vi "Actor Core.vi"(8 "error in":errorcluster, 11 "Nested in":refnum<class "UI Actor.lvclass">) -> (0 "error out":errorcluster, 3 "Actor out":refnum<class "Actor.lvclass">)   [LabVIEW 2020, in "UI Actor.lvlib" / "UI Actor.lvclass"]
doc: "(<B>Filename</B>: Actor Framework.lvlib:Actor.lvclass:Actor Core.vi)\n\nReceives messages to the actor, reacts to them, and initiates any error handling that may shut the actor down.\n\nDescendant classes may override this VI to append parallel tasks for the actor to complete while it handles messages. Overrides use the Call Parent Method node."
uses:
  UI Actor.lvclass
  <vilib>/ActorFramework/Actor/Actor.lvclass
  <vilib>/ActorFramework/Stop Msg/Stop Msg.lvclass
  Sub Panel Actor.lvclass
  C:/Program Files (x86)/National Instruments/LabVIEW 2020/vi.lib/ActorFramework/Actor/Actor.lvclass
  C:/Users/eddiews/Documents/Git Hub Repositorios/VendingMachine_ActorFramework/UI Actor.lvclass
  C:/Users/eddiews/Documents/Git Hub Repositorios/VendingMachine_ActorFramework/Sub Panel Actor.lvclass
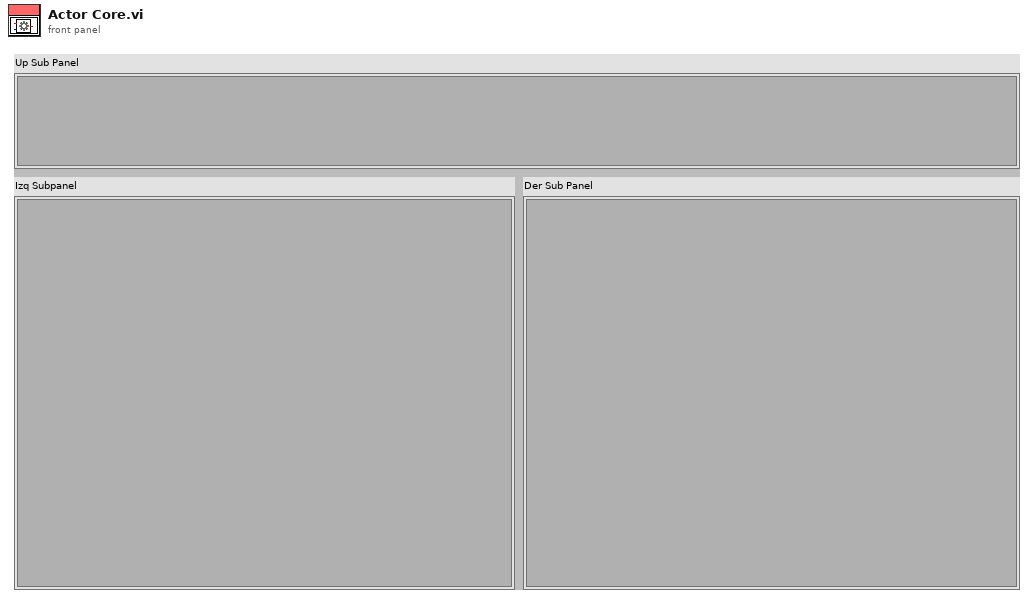
[diagram p1: front panel]
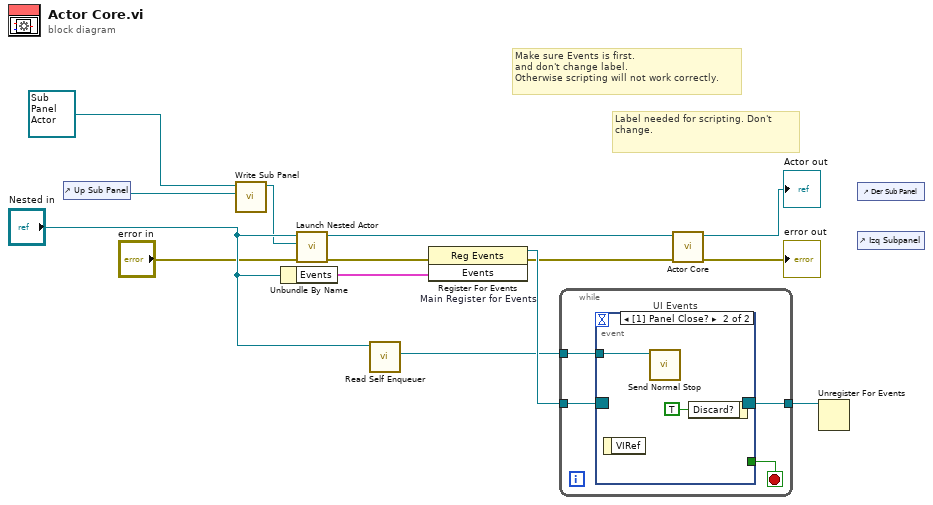
[diagram p0: block diagram]
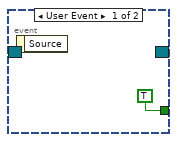
[diagram p2: hidden frame]
diagram:
  # "Label needed for scripting. Don't change."
  # "Make sure Events is first.\nand don't change label.\nOtherwise scripting will not work correctly."
  n1 = control-ref of="Up Sub Panel"() -> (w1:refnum<vi>)
  n2 = call "Write Sub Panel.vi"("Sub Panel"=w1, "Sub Panel Actor in"=refnum<class "Sub Panel Actor.lvclass"> refnum ("Sub Panel Actor.lvlib:Sub Panel Actor.lvclass")) -> ("Sub Panel Actor out"=w4:refnum<class "Sub Panel Actor.lvclass">)  [unwired: 8 in, 1 out]
  n3 = Unbundle By Name("Nested in") -> ("Events"=w11:cluster{"Stop":refnum<user-event>})
  n4 = call <vilib>:"Launch Nested Actor.vi"("error in (no error)"="error in", "Nested Actor"=w4, "Caller Actor in"="Nested in") -> ("error out"=w3:errorcluster, "Caller Actor out"=w6:refnum<class "UI Actor.lvclass">)  [unwired: 6 in, 1 out]
  n5 = call <vilib>:"Read Self Enqueuer.vi"("Actor"="Nested in") -> ("Self Enqueuer"=w9:refnum<class "Message Enqueuer.lvclass">)  [unwired: 10 in]
  n6 = register-events "Main Register for Events"(error in=w3, w11) -> (reference out=w12:refnum<event-registration>, error out=w8:errorcluster)  [unwired: 1 in]
  n7 = while {
    tunnel: w12 -> [w18]
    tunnel: [w16] -> w10
    tunnel: w9 -> [w15]
    stop <- w17 stop-if-true
    n8 = event "UI Events" shown="[1] Panel Close?" {
      selector: w18 -> [_ _]
      dyn-events: [_ _] -> w16
      timeout: _ -> [_ _]
      tunnel: [TRUE _] -> w17
      tunnel: w15 -> [_ w20]
      event User Event {
        n9 = event-data() -> ()  [unwired: 1 in, 1 out]
      }
      event Panel Close? {
        n10 = event-data() -> ()  [unwired: 1 in, 1 out]
        n11 = call <vilib>:"Send Normal Stop.vi"("Message Enqueuer"=w20) -> ()  [unwired: 10 in, 1 out]
        n12 = event-data("Discard?"=TRUE) -> ()  [unwired: 1 in, 1 out]
      }
    }
  }
  n13 = call-parent "Actor Core.vi"("error in"=w8, "Actor in"=w6) -> ("error out"=→"error out":errorcluster, "Actor out"=→"Actor out":refnum<class "Actor.lvclass">)  [unwired: 8 in]
  n14 = Unregister For Events(event registration refnum=w10) -> ()  [unwired: 1 in, 1 out]
  n15 = control-ref of="Der Sub Panel"() -> ()  [unwired: 1 out]
  n16 = control-ref of="Izq Subpanel"() -> ()  [unwired: 1 out]
